vi "Gui_Set_Rings_Refs.vi"(8 "error in (no error)":errorcluster, 9 "Path":path, 10 "EXPERIMENT Inputs":T1={"Setup"="", "Date"="", "User Name"="", "Comment"="", "Experiment Procedures"=[], "Chemical Source"="", "Sample Components"=[], "Species"=[], "Laser 1"={"Used"=TRUE, "Name"="Spectroscopy", "Wavelength"=1000.0, "Energy"=25.0}, "Laser 2"={"Used"=TRUE, "Name"="Spectroscopy", "Wavelength"=1000.0, "Energy"=25.0}, "Laser 3"={"Used"=TRUE, "Name"="Spectroscopy", "Wavelength"=1000.0, "Energy"=25.0}, "Laser 4"={"Used"=TRUE, "Name"="Spectroscopy", "Wavelength"=1000.0, "Energy"=25.0}, "Laser 5"={"Used"=TRUE, "Name"="Spectroscopy", "Wavelength"=1000.0, "Energy"=25.0}, "Lamp 1"={"Used"=TRUE, "Name"="Spectroscopy", "Wavelength"=1000.0, "Attenuation"=25.0}, "Lamp 2"={"Used"=TRUE, "Name"="Spectroscopy", "Wavelength"=1000.0, "Attenuation"=25.0}, "Gas 1"={"Used"=TRUE, "Name"="Spectroscopy", "Pressure"=1000.0}, "Gas 2"={"Used"=TRUE, "Name"="Spectroscopy", "Pressure"=1000.0}, "Gas 3"={"Used"=TRUE, "Name"="Spectroscopy", "Pressure"=1000.0}, "Gas 4"={"Used"=TRUE, "Name"="Spectroscopy", "Pressure"=1000.0}, "Gas 5"={"Used"=TRUE, "Name"="Spectroscopy", "Pressure"=1000.0}}, 11 "Rings Refs":refnum<vi>[](array[refnum])) -> (0 "error out":errorcluster caption="sortie d'erreur", 3 "Rings Refs out":refnum<vi>[](array[refnum]))   [LabVIEW 2020]
doc: "This VI fills many rings with values read from several text files.\nA table of references to the rings is used."
uses:
  controls/EXPERIMENT_Inputs.ctl
  controls/LASER_Inputs.ctl
  controls/LAMP_Inputs.ctl
  controls/GAS_Inputs.ctl
panel:
  # "Lasers"
  # "nm"
  # "mJ"
  # "Lamps"
  # "nm"
  # "dB"
  # "Gas"
  # "bar"
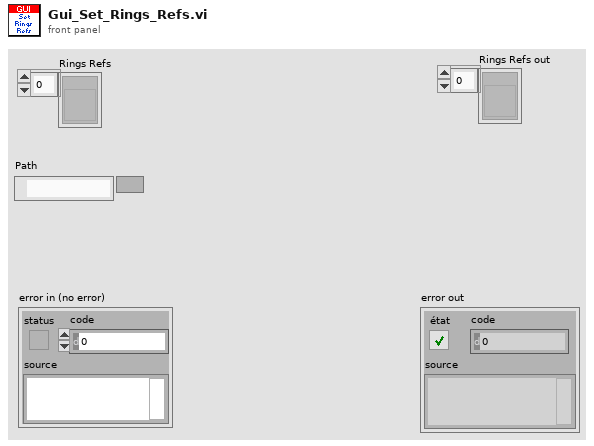
[diagram p1: front panel]
types:
  T1 = typedef "EXPERIMENT_Inputs.ctl" = cluster{"Setup":string, "Date":string, "User Name":string, "Comment":string, "Experiment Procedures":string[], "Chemical Source":string, "Sample Components":string[], "Species":string[], "Laser 1":T2, "Laser 2":T2, "Laser 3":T2, "Laser 4":T2, "Laser 5":T2, "Lamp 1":T3, "Lamp 2":T3, "Gas 1":T4, "Gas 2":T4, "Gas 3":T4, "Gas 4":T4, "Gas 5":T4}
  T2 = typedef "LASER_Inputs.ctl" = cluster{"Used":bool, "Name":string, "Wavelength":dbl, "Energy":dbl}
  T3 = typedef "LAMP_Inputs.ctl" = cluster{"Used":bool, "Name":string, "Wavelength":dbl, "Attenuation":dbl}
  T4 = typedef "GAS_Inputs.ctl" = cluster{"Used":bool, "Name":string, "Pressure":dbl}
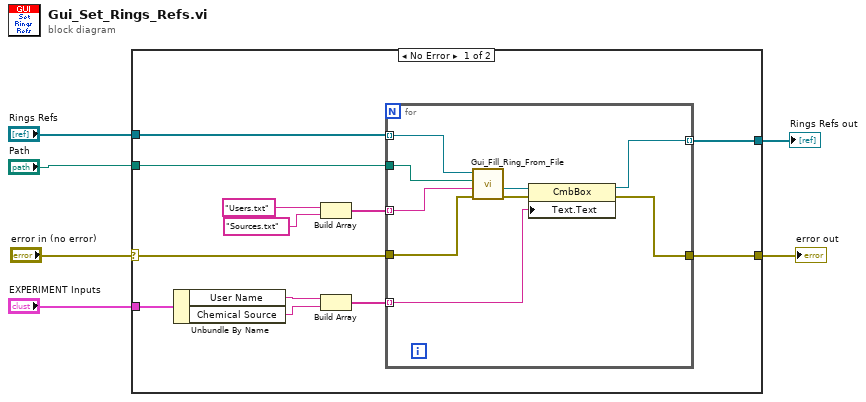
[diagram p0: block diagram]
diagram:
  n1 = case shown="No Error" "error in (no error)" {
    selector: "error in (no error)" -> [w18 w29]
    tunnel: [w12 w29] -> w6
    tunnel: "Rings Refs" -> [w14 w28]
    tunnel: [w13 w28] -> w1
    tunnel: "Path" -> [w11 _]
    tunnel: "EXPERIMENT Inputs" -> [w10 _]
    frame No Error {
      n2 = Unbundle By Name(w10) -> ("User Name"=w16:string, "Chemical Source"=w17:string)
      n3 = Build Array("Users.txt", "Sources.txt") -> (w7:string[])
      n4 = Build Array(w16, w17) -> (w15:string[])
      n5 = for {
        tunnel: w15 -> [w23] mode=indexing
        tunnel: w14 -> [w21] mode=indexing
        tunnel: [w27] -> w13 mode=indexing
        tunnel: w18 -> [w20]
        tunnel: [w26] -> w12
        tunnel: w11 -> [w25]
        tunnel: w7 -> [w22] mode=indexing
        n6 = call "Gui_Fill_Ring_From_File.vi"("error in (no error)"=w20, "Resource Name"=w22, "Resource Path"=w25, "Refnum ChneDér"=w21) -> ("error out"=w24:errorcluster, "Refnum ChneDér out"=w19:refnum<vi>)  [unwired: 4 in, 2 out]
        n7 = property class="CmbBox"(reference=w19, error in=w24, "Text.Text"=w23) -> (reference out=w27:refnum<vi>, error out=w26:errorcluster)
      }
    }
    frame Error {
    }
  }
  "error out" <- w6
  "Rings Refs out" <- w1
